vi "Handle.vi"(8 "error in (no error)":errorcluster, 10 "Zero Timeout Message Handler in":refnum<class "Zero Timeout Message Handler.lvclass">, 11 "Message in":refnum<class "Set PID Gains Msg.lvclass">) -> (0 "error out":errorcluster, 2 "Zero Timeout Message Handler out":refnum<class "Zero Timeout Message Handler.lvclass">)   [LabVIEW 2024, in "PID Loop.lvlib" / "Set PID Gains Msg.lvclass"]
uses:
  src/Zero Timeout Message Handler/Zero Timeout Message Handler/Zero Timeout Message Handler.lvclass
  Set PID Gains Msg.lvclass
  Set PID Gains Msg.lvclass/Set PID Gains Msg.ctl
  PID Loop.lvclass
  C:/Users/uspoaotto/OneDrive - Oregon Tool/Desktop/working copies/zeroTimeoutMessageHandler/src/Zero Timeout Message Handler/Zero Timeout Message Handler/Zero Timeout Message Handler.lvclass
  C:/Users/uspoaotto/OneDrive - Oregon Tool/Desktop/working copies/zeroTimeoutMessageHandler/samples/PID Controller/PID Loop/PID Loop/PID Loop.lvclass
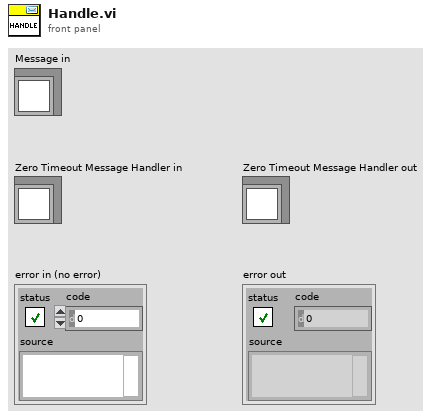
[diagram p1: front panel]
types:
  T1 = cluster{"proportional gain (Kc)":dbl, "integral time (Ti, min)":dbl, "derivative time (Td, min)":dbl}
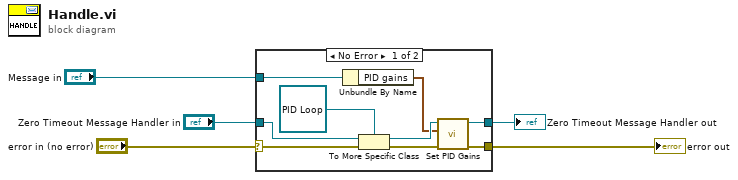
[diagram p0: block diagram]
diagram:
  n1 = case shown="No Error" "error in (no error)" {
    selector: "error in (no error)" -> [w10 w15]
    tunnel: "Zero Timeout Message Handler in" -> [w14 w16]
    tunnel: "Message in" -> [w9 _]
    tunnel: [w7 w16] -> w2
    tunnel: [w6 w15] -> w1
    frame No Error {
      n2 = Unbundle By Name(w9) -> ("PID gains"=w8:T1)
      n3 = To More Specific Class(target class=refnum<class "PID Loop.lvclass"> refnum ("PID Loop.lvlib:PID Loop.lvclass"), reference=w14, error in=w10) -> (specific class reference=w12:refnum<class "PID Loop.lvclass">, error out=w11:errorcluster)
      n4 = call-dynamic "Set PID Gains.vi"("error in (no error)"=w11, "PID gains"=w8, "PID Loop in"=w12) -> ("error out"=w6:errorcluster, "PID Loop out"=w7:refnum<class "PID Loop.lvclass">)  [unwired: 7 in]
    }
    frame Error {
    }
  }
  "error out" <- w1
  "Zero Timeout Message Handler out" <- w2
